vi "Get Specific DAC.vi"(6 "DAC Class Name":string, 8 "error in":errorcluster, 11 "Generic Test Stand in":refnum<class "Generic Test Stand.lvclass">) -> (0 "error out":errorcluster, 2 "DAC":refnum<class "DAC.lvclass">, 3 "Generic Test Stand out":refnum<class "Generic Test Stand.lvclass">)   [LabVIEW 2019, in "Generic Test Stand.lvclass"]
uses:
  Generic Test Stand.lvclass
  DAC/DAC.lvclass
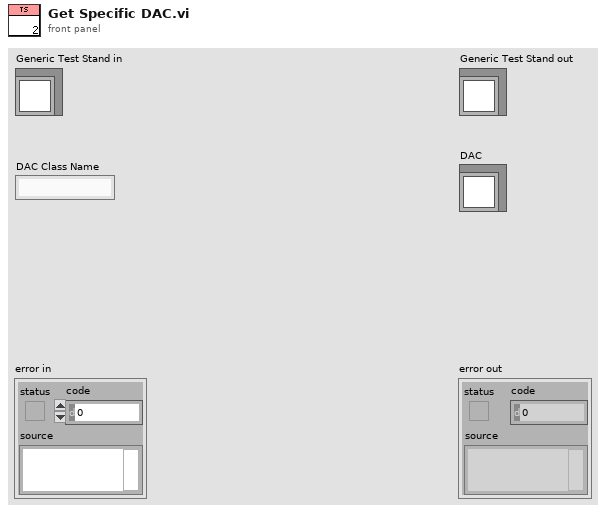
[diagram p1: front panel]
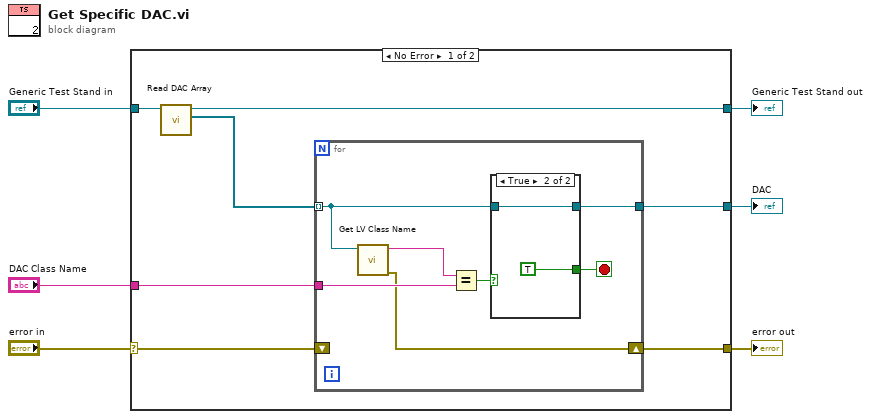
[diagram p0: block diagram]
diagram:
  n1 = case shown="No Error" "error in" {
    selector: "error in" -> [w9 w25]
    tunnel: [w8 w25] -> w5
    tunnel: [w11 w24] -> w3
    tunnel: "Generic Test Stand in" -> [w12 w24]
    tunnel: "DAC Class Name" -> [w10 _]
    tunnel: [w7 _] -> w1
    frame No Error {
      n2 = call "Read DAC Array.vi"("Generic Test Stand in"=w12) -> ("DAC Array"=w13:refnum<class "DAC.lvclass">[], "Generic Test Stand out"=w11:refnum<class "Generic Test Stand.lvclass">)  [unwired: 8 in, 1 out]
      n3 = for {
        tunnel: w13 -> [w18] mode=indexing
        tunnel: w10 -> [w17]
        tunnel: [w16] -> w7
        shift-right: [w14] -> w8
        shift-left: w9 -> [_]
        stop <- w15 stop-if-true
        n4 = call <vilib>:"Get LV Class Name.vi"("object"=w18) -> ("error out"=w14:errorcluster, "class name"=w20:string)  [unwired: 9 in]
        n5 = Equal?(x=w20, y=w17) -> (x = y?=w19:bool)
        n6 = case shown="True" w19 {
          tunnel: w18 -> [w21 w23]
          tunnel: [w21 w23] -> w16
          tunnel: [_ TRUE] -> w15
          frame False {
          }
          frame True {
          }
        }
      }
    }
    frame Error {
    }
  }
  "error out" <- w5
  "Generic Test Stand out" <- w3
  "DAC" <- w1
